vi "InitAction.vi"(6 "InstrumentName":string, 7 "VisaRessIn":refnum<visa-resource-name>, 8 "error in (no error)":errorcluster caption="entrée d'erreur (pas d'erreur)", 9 "FirstClassInst":bool, 10 "Function":string, 11 "GenData In":refnum<class "LeafMagnetometer.lvclass"> caption="DNL_LabVIEW Object in") -> (0 "error out":errorcluster caption="sortie d'erreur", 3 "GenData Out":refnum<class "LeafMagnetometer.lvclass"> caption="DNL_LabVIEW Object out")   [LabVIEW 2012, in "LeafMagnetometer.lvclass"]
uses:
  LeafMagnetometer.lvclass
  LeafMagnetometer_Func.ctl
  LeafMagnetometer.lvclass/LeafMagnetometer.ctl
panel:
  in  "DefaultDev_Func":T1
  out "VisaRessOut":refnum<visa-resource-name>
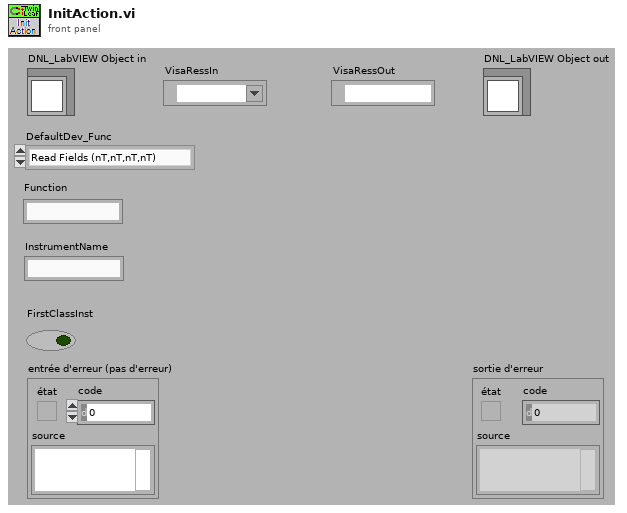
[diagram p1: front panel]
types:
  T1 = typedef "LeafMagnetometer.lvclass/LeafMagnetometer_Func.ctl" = enum16{"Read Fields (nT,nT,nT,nT)", "Read AVM Fields (nT)"}
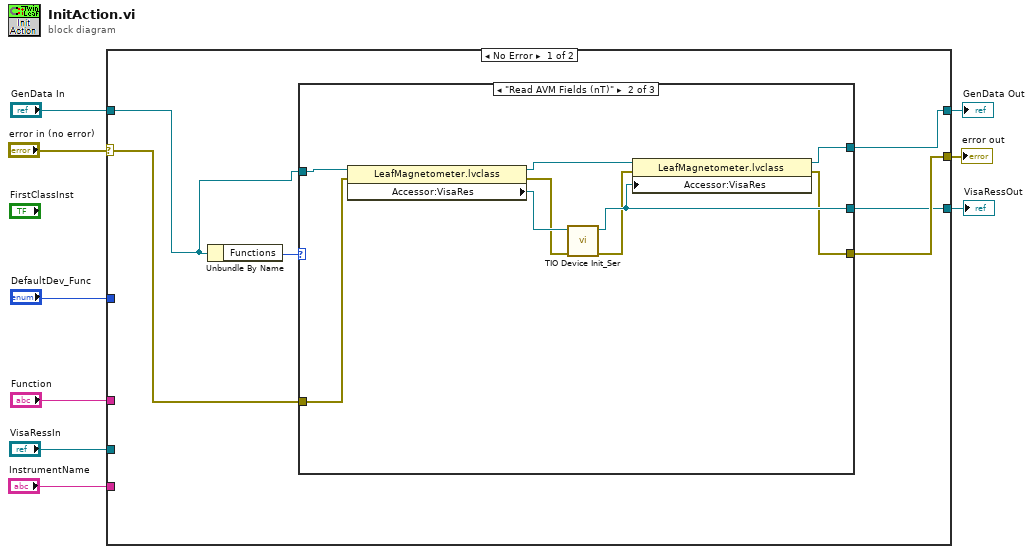
[diagram p0: block diagram]
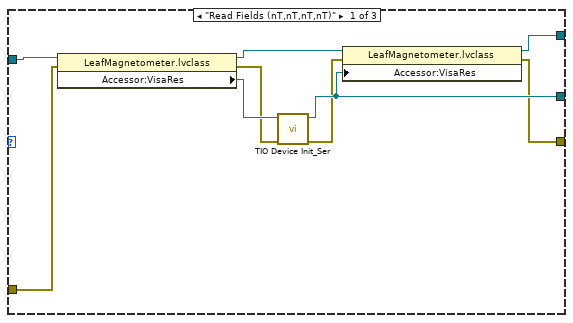
[diagram p2: hidden frame]
diagram:
  n1 = case shown="No Error" "error in (no error)" {
    selector: "error in (no error)" -> [w13 w38]
    tunnel: [w12 w38] -> w8
    tunnel: "GenData In" -> [w14 w37]
    tunnel: [w10 w37] -> w6
    tunnel: "DefaultDev_Func" -> [_ _]
    tunnel: "Function" -> [_ _]
    tunnel: "InstrumentName" -> [_ _]
    tunnel: [w11 w36] -> w2
    tunnel: "VisaRessIn" -> [_ w36]
    frame No Error {
      n2 = Unbundle By Name(w14) -> ("Functions"=w15:T1)
      n3 = case shown="\"Read AVM Fields (nT)\"" w15 {
        tunnel: w14 -> [w24 w33 w34]
        tunnel: w13 -> [w22 w31 w35]
        tunnel: [w16 w25 w35] -> w12
        tunnel: [w18 w27 _] -> w11
        tunnel: [w19 w28 w34] -> w10
        frame "Read Fields (nT,nT,nT,nT)" {
          n4 = property class="LeafMagnetometer.lvclass"(reference=w24, error in=w22) -> (reference out=w20:refnum<class "LeafMagnetometer.lvclass">, error out=w21:errorcluster, "Accessor:VisaRes"=w23:refnum<visa-resource-name>)
          n5 = call <userlib>:"TIO Device Init_Ser.vi"("error in (no error)"=w21, "Nom de ressource VISA"=w23) -> ("error out"=w17:errorcluster, "Nom de ressource VISA Out"=w18:refnum<visa-resource-name>)  [unwired: 6 in, 2 out]
          n6 = property class="LeafMagnetometer.lvclass"(reference=w20, error in=w17, "Accessor:VisaRes"=w18) -> (reference out=w19:refnum<class "LeafMagnetometer.lvclass">, error out=w16:errorcluster)
        }
        frame "Read AVM Fields (nT)" {
          n7 = property class="LeafMagnetometer.lvclass"(reference=w33, error in=w31) -> (reference out=w29:refnum<class "LeafMagnetometer.lvclass">, error out=w30:errorcluster, "Accessor:VisaRes"=w32:refnum<visa-resource-name>)
          n8 = call <userlib>:"TIO Device Init_Ser.vi"("error in (no error)"=w30, "Nom de ressource VISA"=w32) -> ("error out"=w26:errorcluster, "Nom de ressource VISA Out"=w27:refnum<visa-resource-name>)  [unwired: 6 in, 2 out]
          n9 = property class="LeafMagnetometer.lvclass"(reference=w29, error in=w26, "Accessor:VisaRes"=w27) -> (reference out=w28:refnum<class "LeafMagnetometer.lvclass">, error out=w25:errorcluster)
        }
        frame Default {
        }
      }
    }
    frame Error {
    }
  }
  "error out" <- w8
  "GenData Out" <- w6
  "VisaRessOut" <- w2
